vi "Get All Property Data.vi"(8 "error in":errorcluster, 11 "Item in":refnum<class "Item.lvclass">) -> (0 "error out":errorcluster, 2 "Properties Data":T2(array[cluster]), 3 "Item out":refnum<class "Item.lvclass">)   [LabVIEW 2024, in "Parser.lvlib" / "Property.lvclass"]
uses:
  Property.lvclass
  Property.lvclass/Property.ctl
  Controls/Property Type.ctl
  Item/Item.lvclass
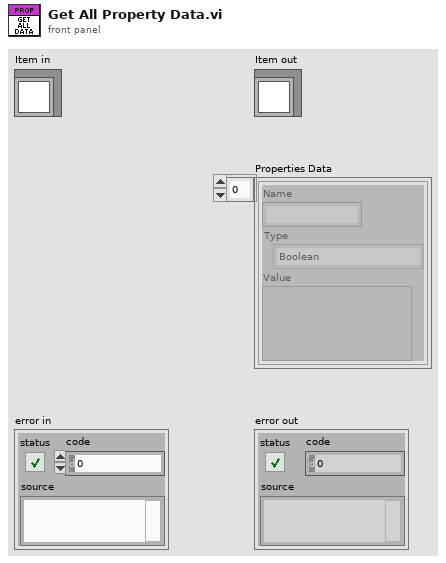
[diagram p1: front panel]
types:
  T1 = typedef "Parser.lvlib/Property.lvclass/Property Type.ctl" = enum16{"Boolean", "Double", "String", "Path", "Dictionary", "DependentFile", "I16", "I32", "I64", "U16", "U32", "U64", "BooleanArray", "DoubleArray", "StringArray", "I16Array", "I32Array", "I64Array", "U16Array", "U32Array", "U64Array", "Variant"}
  T2 = cluster{"Name":string, "Type":T1, "Value":variant}[]
  T3 = cluster{"Name":string, "Type":T1, "Value":variant}
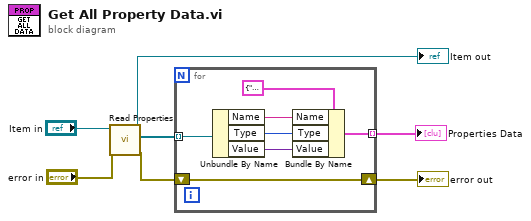
[diagram p0: block diagram]
diagram:
  n1 = call "Read Properties.vi"("error in"="error in", "Item in"="Item in") -> ("error out"=w6:errorcluster, "Properties"=w2:refnum<class "Property.lvclass">[], "Item out"=→"Item out":refnum<class "Item.lvclass">)  [unwired: 7 in]
  n2 = for {
    tunnel: w2 -> [w13] mode=indexing
    tunnel: [w8] -> w4 mode=indexing
    shift-right: [w14] -> w5
    shift-left: w6 -> [w14]
    n3 = Unbundle By Name(w13) -> ("Name"=w12:string, "Type"=w10:T1, "Value"=w9:variant)
    n4 = Bundle By Name(cluster=T3 {"Name"="", "Type"=enum."Boolean", "Value"=variant}, "Name"=w12, "Type"=w10, "Value"=w9) -> (w8:T3)
  }
  "error out" <- w5
  "Properties Data" <- w4
